vi "Coverate Include File Path From Test Cases.vi"(11 "Test Case Classes":path[](array[path])) -> (3 "appended path":path)   [LabVIEW 2020, in "Coverage Report.lvclass"]
uses:
  Coverage Report.lvclass
  Coverage Report.lvclass/Coverage Report.ctl
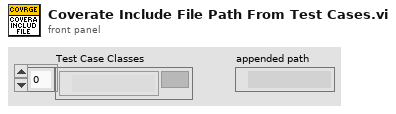
[diagram p1: front panel]
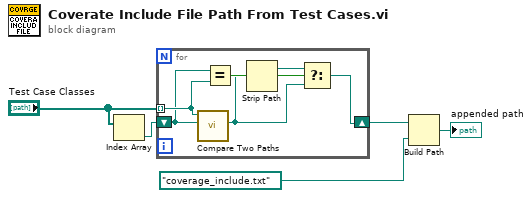
[diagram p0: block diagram]
diagram:
  n1 = Index Array(array="Test Case Classes") -> (element=w2:path)  [unwired: 1 in]
  n2 = for {
    tunnel: "Test Case Classes" -> [w11] mode=indexing
    shift-right: [w8] -> w3
    shift-left: w2 -> [w10]
    n3 = call <vilib>:"Compare Two Paths.vi"("Path 2"=w10, "Path 1"=w11) -> ("Common Path"=w7:path)  [unwired: 6 in, 3 out]
    n4 = Equal?(x=w10, y=w11) -> (x = y?=w9:bool)
    n5 = Strip Path(path=w7) -> (stripped path=w6:path)  [unwired: 1 out]
    n6 = Select(t=w6, s=w9, f=w7) -> (s? t:f=w8:path)
  }
  n7 = Build Path(base path=w3, name or relative path=path "coverage_include.txt") -> (appended path=→"appended path":path)
